vi "Increment Model Data.vi"(6 "Publish Time (Use Current Time)":timestamp, 8 "error in (no error)":errorcluster, 9 "Numeric Type":variant, 10 "Datum Name":string, 11 "IModel in":refnum<class "IModel.lvclass">) -> (0 "error out":errorcluster, 3 "IModel out":refnum<class "IModel.lvclass">)   [LabVIEW 2015, in "IModel.lvlib" / "IModel.lvclass"]
doc: "Publish a datum (value) to the mediator bus. Published data are observable by any actor with access to the mediated bus."
uses:
  IModel.lvclass
  <vilib>/ActorFramework/Actor/Actor.lvclass/Actor.ctl
  <vilib>/ActorFramework/Message Enqueuer/Message Enqueuer.lvclass/Message Enqueuer.ctl
  IModel.lvclass/IModel.ctl
  PublicationPolicy/IncrementValuePublication/IncrementValuePublication.lvclass
  IMediator/PublishRequest/PublishRequest.lvclass/PublishRequest.ctl
  IMediator/MutexedPublishRequest/MutexedPublishRequest.lvclass/MutexedPublishRequest.ctl
  AbstractMessages/PreAddressedMsg/PreAddressedMsg.lvclass/PreAddressedMsg.ctl
  IMediator/IMediator Messages/Publish Msg/Publish Msg.lvclass/Publish Msg.ctl
  <vilib>/ActorFramework/Actor/Read Self Enqueuer.vi
  <vilib>/ActorFramework/Message Enqueuer/Enqueue.vi
  AbstractMessages/PreAddressedMsg/Read Return Address.vi
  IMediator/PublishRequest/Write Publish Request Data.vi
  <vilib>/ActorFramework/Message Enqueuer/Init from Existing Queue.vi
  <vilib>/ActorFramework/Message Priority Queue/Priority Enqueue.vi
  IMediator/MutexedPublishRequest/MutexedPublishRequest.lvclass
  IMediator/ITransport/ITransport.lvclass
  <vilib>/ActorFramework/Message Enqueuer/Message Enqueuer.lvclass
  <vilib>/ErrorRing/Error Ring.xnode
  IMediator/IMediator Messages/Publish Msg/Publish Msg.lvclass
  IObserver/IObserver/IObserver.lvclass
  <vilib>/Utility/Data Type/NI_Data Type.lvlib
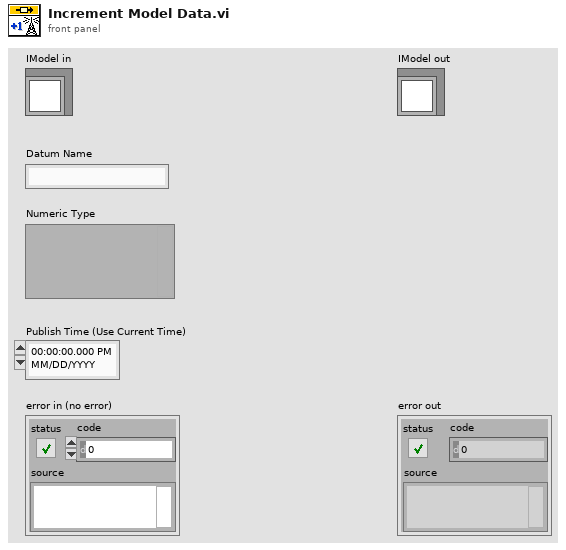
[diagram p1: front panel]
types:
  T1 = typedef "NI_Data Type.lvlib/Data Type.ctl" = enum8{"Invalid Type", "Void", "I8", "I16", "I32", "I64", "U8", "U16", "U32", "U64", "Single Float", "Double Float", "Extended Float", "Single Complex", "Double Complex", "Extended Complex", "Enum U8", "Enum U16", "Enum U32", "Enum U64", "Single Float With Unit", "Double Float With Unit", "Extended Float With Unit", "Single Complex with Unit", "Double Complex with Unit", "Extended Complex with Unit", "Boolean", "String", "Path", "Picture", "Tag", "Array", "Cluster", "Variant", "LV Variant", "Waveform", "Timestamp", "Digital Waveform", "Digital Data", "ExpressData", "Refnum", "External Data", "VI", "Poly VI", "LabVIEW Class Instance", "Fixed Point"}
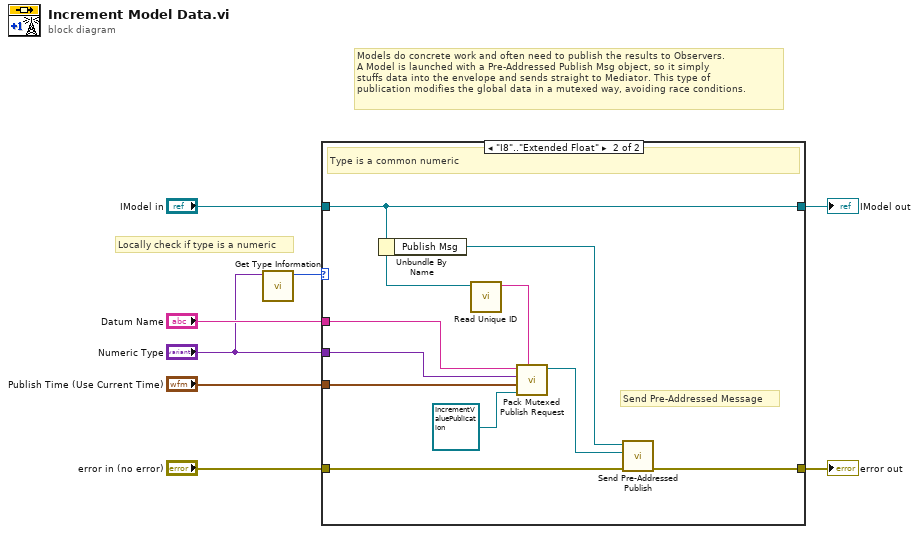
[diagram p0: block diagram]
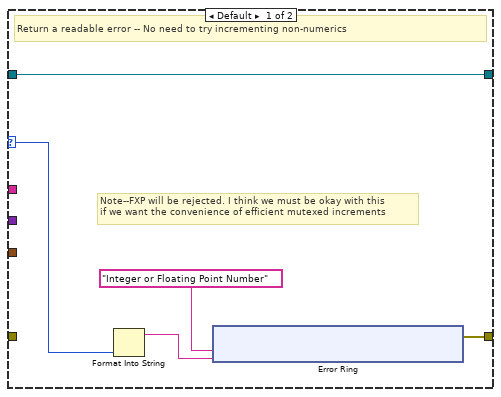
[diagram p2: hidden frame]
diagram:
  # "Locally check if type is a numeric"
  # "Models do concrete work and often need to publish the results to Observers.\nA Model is launched with a Pre-Addressed Publish Msg object, so it simply\nstuffs data into the envelope and sends straight to Mediator. This type of\npublication modifies the global data in a mutexed way, avoiding race conditions."
  n1 = call <vilib>:"Get Type Information.vi"("Variant"="Numeric Type") -> ("Type"=w1:T1)  [unwired: 6 in, 4 out]
  n2 = case shown="\"I8\"..\"Extended Float\"" w1 {
    selector: w1 -> [w9 _]
    tunnel: "error in (no error)" -> [_ w28]
    tunnel: [w12 w27] -> w7
    tunnel: "IModel in" -> [w13 w20]
    tunnel: "Datum Name" -> [_ w26]
    tunnel: "Numeric Type" -> [_ w25]
    tunnel: "Publish Time (Use Current Time)" -> [_ w24]
    tunnel: [w13 w20] -> w3
    frame Default {
      # "Note--FXP will be rejected. I think we must be okay with this\nif we want the convenience of efficient mutexed increments"
      # "Return a readable error -- No need to try incrementing non-numerics"
      n3 = Format Into String(w9) -> (resulting string=w10:string)  [unwired: 3 in, 1 out]
      n4 = xnode "Error Ring"("parameter 0"="Integer or Floating Point Number", "parameter 1"=w10) -> ("error out"=w12:errorcluster)
    }
    frame "I8".."Extended Float" {
      # "Send Pre-Addressed Message"
      # "Type is a common numeric"
      n5 = Unbundle By Name(w20) -> ("Publish Msg"=w29:refnum<class "Publish Msg.lvclass">)
      n6 = call "Read Unique ID.vi"("IObserver In"=w20) -> ("Unique ID"=w22:string)  [unwired: 10 in]
      n7 = call "Pack Mutexed Publish Request.vi"("Publisher ID"=w22, "PublicationPolicy"=refnum<class "IncrementValuePublication.lvclass"> refnum ("PublicationPolicy.lvlib:IncrementValuePublication.lvclass"), "Publish Time (Use Current Time)"=w24, "Datum Value or Type"=w25, "Datum Name"=w26) -> ("MutexedPublishRequest Out"=w23:refnum<class "MutexedPublishRequest.lvclass">)  [unwired: 6 in]
      n8 = call "Send Pre-Addressed Publish.vi"("error in (no error)"=w28, "PublishRequest"=w23, "Publish Message"=w29) -> ("error out"=w27:errorcluster)  [unwired: 8 in]
    }
  }
  "IModel out" <- w3
  "error out" <- w7
